vi "Calculate TOP (Phase Correct Mode).vi"(9 "Requested Frequency (Hz)":dbl, 10 "Clock Divisor":u32, 11 "Base Clock Frequency (Hz)":dbl) -> (2 "TOP":dbl, 3 "Remainder?":bool)   [LabVIEW 2021]
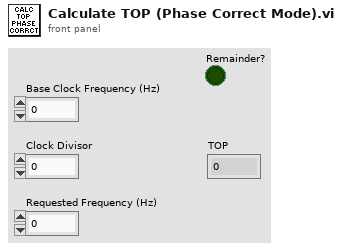
[diagram p1: front panel]
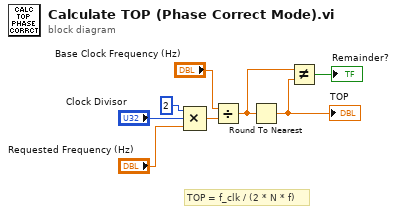
[diagram p0: block diagram]
diagram:
  # "TOP = f_clk / (2 * N * f)"
  n1 = Compound Arithmetic op=MULTIPLY(2, "Clock Divisor", "Requested Frequency (Hz)") -> (w7:dbl)
  n2 = Divide(x="Base Clock Frequency (Hz)", y=w7) -> (x/y=w1:dbl)
  n3 = Round To Nearest(number=w1) -> (nearest integer value=w2:dbl)
  "TOP" <- w2
  n4 = Not Equal?(x=w1, y=w2) -> (x != y?=→"Remainder?":bool)
